vi "Link Control References.vi"(8 "error in (no error)":errorcluster, 10 "Control References":T1[](array[typedef]), 11 "Fault Monitor in":refnum<class "Fault Monitor.lvclass">) -> (0 "error out":errorcluster, 3 "Fault Monitor out":refnum<class "Fault Monitor.lvclass">)   [LabVIEW 2023, in "Fault Monitor.lvlib" / "Fault Monitor.lvclass"]
doc: "<b> Link Control References </b>\n<b> Engine Level </b>\nThis is the base abstraction layer. The purpose of this method is to link the control references to the class private data."
uses:
  Library/Fault Monitor.lvclass
  builds/Framework/Engine.lvlibp/Engine/Custom Controls/Control Reference.ctl
  Library/Fault Monitor.lvclass/Fault Monitor.ctl
  builds/Framework/Engine.lvlibp/Engine/Library/Engine.lvclass
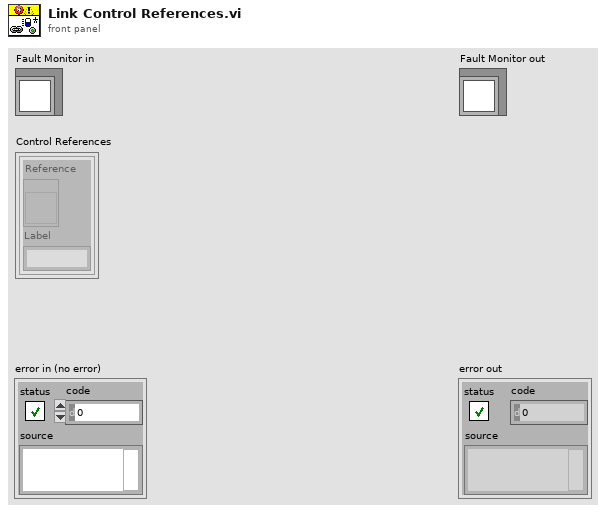
[diagram p1: front panel]
types:
  T1 = typedef "Engine.lvlibp/Engine.lvclass/Control Reference.ctl" = cluster{"Reference":refnum<vi>, "Label":string}
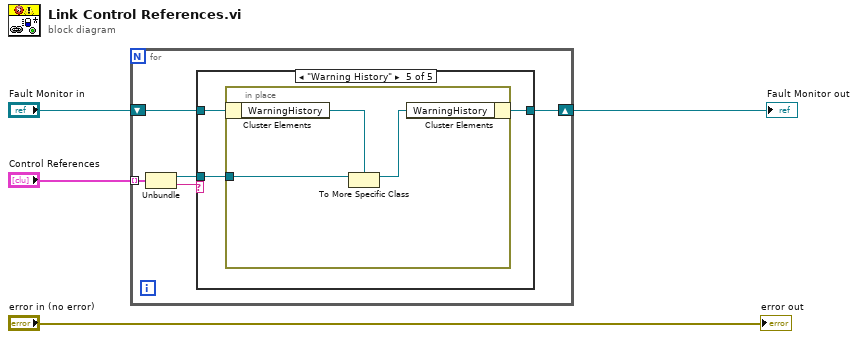
[diagram p0: block diagram]
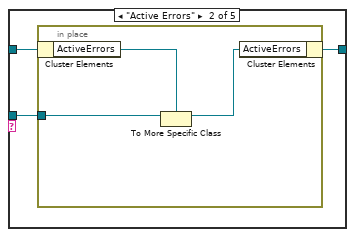
[diagram p3: hidden frame]
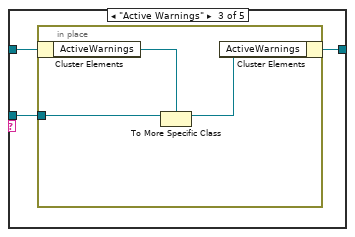
[diagram p4: hidden frame]
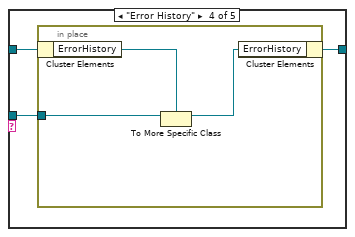
[diagram p5: hidden frame]
diagram:
  n1 = for {
    tunnel: "Control References" -> [w9] mode=indexing
    shift-right: [w5] -> w1
    shift-left: "Fault Monitor in" -> [w6]
    n2 = Unbundle(w9) -> ("Reference"=w7:refnum<vi>, "Label"=w8:string)
    n3 = case shown="\"Warning History\"" w8 {
      tunnel: w7 -> [_ w12 w18 w24 w30]
      tunnel: w6 -> [w10 w13 w19 w25 w31]
      tunnel: [w10 w11 w17 w23 w29] -> w5
      frame "False", Default {
      }
      frame "Active Errors" {
        n4 = in-place {
          in-place-border: w12 -> [w15]
          n5 = in-place-cluster #1(w13) -> ("ActiveErrors"=w16:refnum<vi>)
          n6 = To More Specific Class(target class=w16, reference=w15) -> (specific class reference=w14:refnum<vi>)  [unwired: 1 in, 1 out]
          n7 = in-place-cluster #1("ActiveErrors"=w14) -> (w11:refnum<class "Fault Monitor.lvclass">)
        }
      }
      frame "Active Warnings" {
        n8 = in-place {
          in-place-border: w18 -> [w21]
          n9 = in-place-cluster #2(w19) -> ("ActiveWarnings"=w22:refnum<vi>)
          n10 = To More Specific Class(target class=w22, reference=w21) -> (specific class reference=w20:refnum<vi>)  [unwired: 1 in, 1 out]
          n11 = in-place-cluster #2("ActiveWarnings"=w20) -> (w17:refnum<class "Fault Monitor.lvclass">)
        }
      }
      frame "Error History" {
        n12 = in-place {
          in-place-border: w24 -> [w27]
          n13 = in-place-cluster #3(w25) -> ("ErrorHistory"=w28:refnum<vi>)
          n14 = To More Specific Class(target class=w28, reference=w27) -> (specific class reference=w26:refnum<vi>)  [unwired: 1 in, 1 out]
          n15 = in-place-cluster #3("ErrorHistory"=w26) -> (w23:refnum<class "Fault Monitor.lvclass">)
        }
      }
      frame "Warning History" {
        n16 = in-place {
          in-place-border: w30 -> [w33]
          n17 = in-place-cluster #4(w31) -> ("WarningHistory"=w34:refnum<vi>)
          n18 = To More Specific Class(target class=w34, reference=w33) -> (specific class reference=w32:refnum<vi>)  [unwired: 1 in, 1 out]
          n19 = in-place-cluster #4("WarningHistory"=w32) -> (w29:refnum<class "Fault Monitor.lvclass">)
        }
      }
    }
  }
  "Fault Monitor out" <- w1
  "error out" <- "error in (no error)"
